vi "From JSON.vi"(8 "Error In":errorcluster, 10 "File Path":path, 11 "object in":refnum<class "Continuous Waveform Acq CFG.lvclass">) -> (0 "Error Out":errorcluster, 3 "object out":refnum<class "Continuous Waveform Acq CFG.lvclass">)   [LabVIEW 2023, in "PXIe-5172 Simulated.lvlib" / "Continuous Waveform Acq CFG.lvclass"]
uses:
  Continuous Waveform Acq CFG.lvclass
  Continuous Waveform Acq CFG.lvclass/Continuous Waveform Acq CFG.ctl
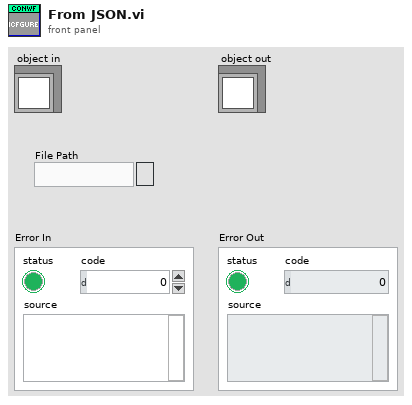
[diagram p1: front panel]
types:
  T1 = cluster{"HW Device Name":string, "Resouce Identifier":string, "Options String":string, "Channels":string, "Vertical Range":dbl, "Vertical Offset":dbl, "Vertical Coupling":i32, "Input Impedance":u32, "Min Sample Rate":dbl}
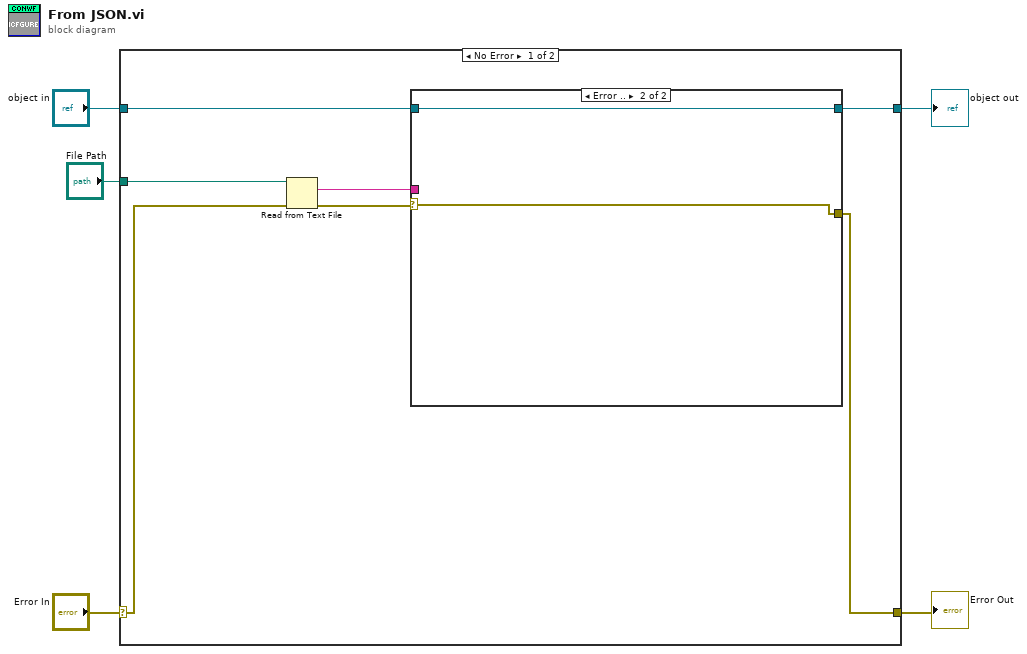
[diagram p0: block diagram]
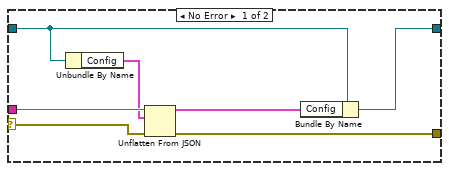
[diagram p2: hidden frame]
diagram:
  n1 = case shown="No Error" "Error In" {
    selector: "Error In" -> [w11 w23]
    tunnel: [w6 w23] -> w4
    tunnel: [w8 w22] -> w2
    tunnel: "object in" -> [w7 w22]
    tunnel: "File Path" -> [w12 _]
    frame No Error {
      n2 = Read from Text File(file (use dialog)=w12, error in=w11) -> (text=w9:string, error out=w10:errorcluster)  [unwired: 2 in, 2 out]
      n3 = case shown="Error .." w10 {
        selector: w10 -> [w13 w20]
        tunnel: w9 -> [w19 _]
        tunnel: [w17 w21] -> w8
        tunnel: w7 -> [w15 w21]
        tunnel: [w14 w20] -> w6
        frame No Error {
          n4 = Unbundle By Name(w15) -> ("Config"=w16:T1)
          n5 = Unflatten From JSON(JSON string=w19, type and defaults=w16, error in (no error)=w13) -> (value=w18:T1, error out=w14:errorcluster)  [unwired: 4 in]
          n6 = Bundle By Name(cluster=w15, "Config"=w18) -> (w17:refnum<class "Continuous Waveform Acq CFG.lvclass">)
        }
        frame Error {
        }
      }
    }
    frame Error {
    }
  }
  "Error Out" <- w4
  "object out" <- w2
